vi "Remove User.vi"(8 "error in (no error)":errorcluster, 10 "Username":string, 11 "UserPwd DB in":refnum<class "UserPwd DB.lvclass">) -> (0 "error out":errorcluster, 2 "found":bool, 3 "UserPwd DB out":refnum<class "UserPwd DB.lvclass">)   [LabVIEW 2016, in "UserPwd DB.lvlib" / "UserPwd DB.lvclass"]
uses:
  <userlib>/Common Components/UserPwd DB/UserPwd DB/UserPwd DB.lvclass
  <userlib>/Common Components/UserPwd DB/UserPwd DB/UserPwd DB.lvclass/UserPwd DB.ctl
  <vilib>/Utility/error.llb/Error Cluster From Error Code.vi
  <vilib>/ErrorRing/Error Ring.xnode
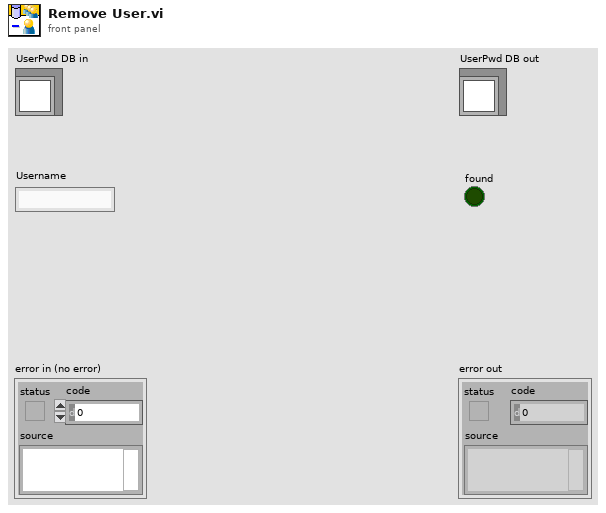
[diagram p1: front panel]
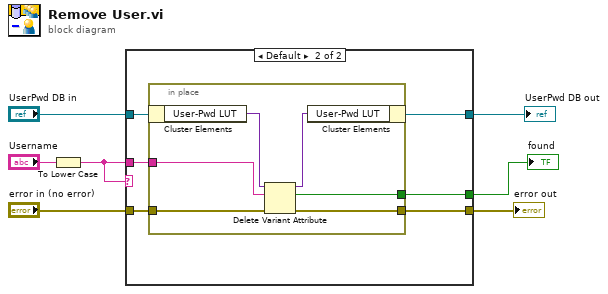
[diagram p0: block diagram]
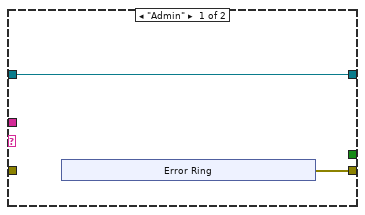
[diagram p2: hidden frame]
diagram:
  n1 = To Lower Case(string="Username") -> (all lower case string=w1:string)
  n2 = case shown="Default" w1 {
    tunnel: "UserPwd DB in" -> [w9 w19]
    tunnel: [w9 w18] -> w6
    tunnel: w1 -> [_ w17]
    tunnel: "error in (no error)" -> [_ w16]
    tunnel: [w8 w15] -> w4
    tunnel: [_ w14] -> w3
    frame "Admin" {
      n3 = xnode "Error Ring"() -> ("error out"=w8:errorcluster)
    }
    frame Default {
      n4 = in-place {
        in-place-border: w17 -> [w23]
        in-place-border: w16 -> [w22]
        in-place-border: [w21] -> w15
        in-place-border: [w20] -> w14
        n5 = in-place-cluster #1(w19) -> ("User-Pwd LUT"=w25:variant)
        n6 = Delete Variant Attribute(4:w22, 6:w23, 7:w25) -> (0:w21:errorcluster, 2:w20:bool, 3:w24:variant)
        n7 = in-place-cluster #1("User-Pwd LUT"=w24) -> (w18:refnum<class "UserPwd DB.lvclass">)
      }
    }
  }
  "error out" <- w4
  "UserPwd DB out" <- w6
  "found" <- w3
